vi "teleop.vi"() -> ()   [LabVIEW 2012, in "Team8953.lvrbt"]
uses:
  Team8953.lvrbt
  <vilib>/NXT/Hardware/Plugins/Tetrix 180 deg Servo/Tetrix180ServoAddress.ctl
  <vilib>/NXT/Hardware/Plugins/Tetrix DC Motor/TetrixDCMotorAddress.ctl
  <vilib>/FTC/FTC Read Controller Packet.vi
  <vilib>/FTC/FTC Read Button States.vi
  <vilib>/NXT/NXTIO Xnodes/NXTIONodeSubVIs/TETRIX IO Move Servos.vi
  <vilib>/FTC/FTC Calculate Drive Power - Arcade Right.vi
  <vilib>/NXT/NXTIO Xnodes/NXTIONodeSubVIs/TETRIX IO Move DC Motors.vi
  <vilib>/NXT/NXTIO Xnodes/NXTIONodeSubVIs/TETRIX IO Check Battery.vi
  <vilib>/NXT/NXTIO Xnodes/NXTIONodeSubVIs/TETRIX IO Stop DC Motors.vi
  <vilib>/NXT/Subs/LVHSConnector.ctl
  <vilib>/NXT/NXTIO Xnodes/AddressXNode/NXTIOAddress.xnode
  <vilib>/NXT/NXTIO Xnodes/NXTIOXNode/NXTIO.xnode
  <vilib>/NXT/LegoClasses/BrickReference/BrickReference.lvclass
panel:
  in  "Drive Power":i8=100 min=-100 max=100
  # "This VI was generated based on your configuration in the Remote Control Editor. You may modify the code as needed for your robot. To test this program for an FTC match, return to the Remote Control Editor, select the \"Run Program\" tab, and choose \"Teleop\"."
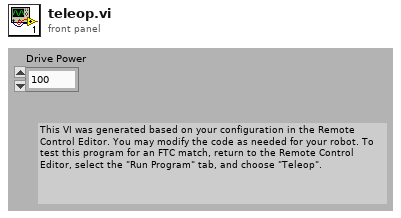
[diagram p1: front panel]
types:
  T1 = typedef "TetrixDCMotorAddress.ctl" = i32
  T2 = cluster{"TetrixDCMotor":T1, "TetrixDCMotor 2":T1}
  T3 = typedef "LVHSConnector.ctl" = refnum<class "BrickReference.lvclass">
  T4 = typedef "FTC ControllerState.ctl" = cluster{"Left X":i8, "Left Y":i8, "Right X":i8, "Right Y":i8, "Button Encoding 9-12":u8, "Button Encoding 1-8":u8, "POV":T5}
  T5 = typedef "FTC POVState.ctl" = i8
  T6 = typedef "FTC ButtonEventType.ctl" = enum16{"Pressed", "Released"}
  T7 = cluster{"Button ID":enum16{"None", "Button 1", "Button 2", "Button 3", "Button 4", "Button 5", "Button 6", "Button 7", "Button 8", "Button 9", "Button 10", "Button 11", "Button 12", "POV Up", "POV Up Right", "POV Right", "POV Down Right", "POV Down", "POV Down Left", "POV Left", "POV Up Left"}, "Event Type":T6}[]
  T8 = enum16{"None", "Button 1", "Button 2", "Button 3", "Button 4", "Button 5", "Button 6", "Button 7", "Button 8", "Button 9", "Button 10", "Button 11", "Button 12", "POV Up", "POV Up Right", "POV Right", "POV Down Right", "POV Down", "POV Down Left", "POV Left", "POV Up Left"}
  T9 = typedef "Tetrix180ServoAddress.ctl" = i32
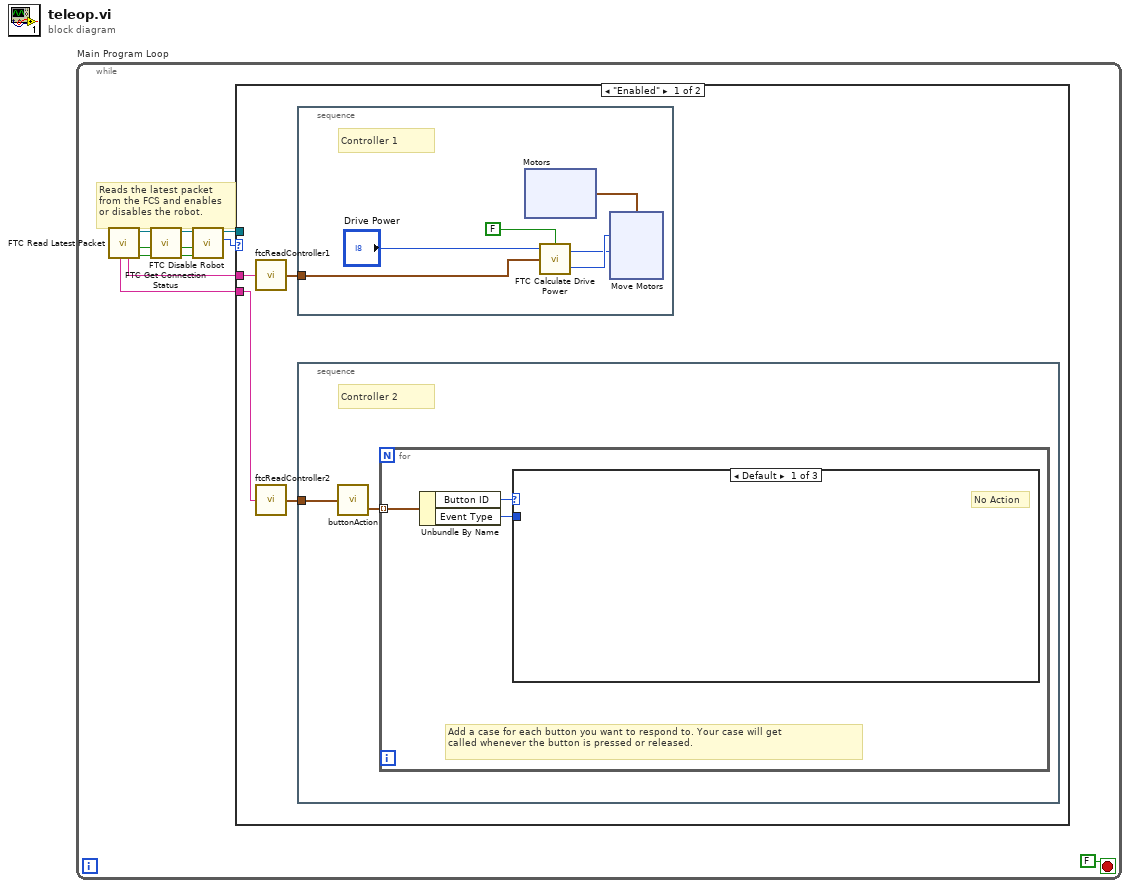
[diagram p0: block diagram]
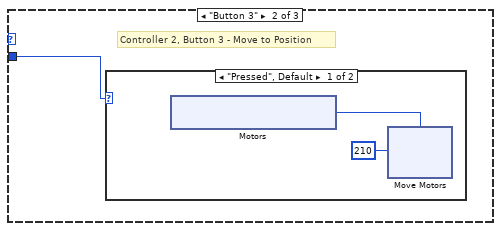
[diagram p2: hidden frame]
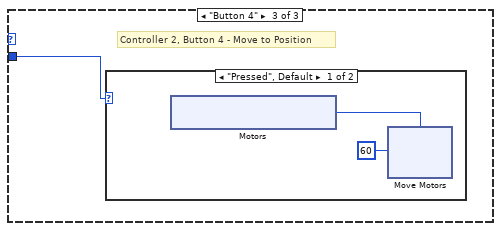
[diagram p4: hidden frame]
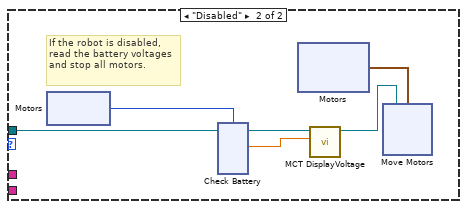
[diagram p6: hidden frame]
diagram:
  n1 = while "Main Program Loop" {
    stop <- FALSE stop-if-true
    # "Reads the latest packet\nfrom the FCS and enables\nor disables the robot."
    n2 = call <vilib>:"FTC Read Latest Packet.vi"() -> ("Packet Received?"=w8:bool, "Stopped?"=w5:bool, "NXT/EV3"=w7:T3, "Controller 1"=w10:string, "Controller 2"=w9:string)  [unwired: 6 in, 1 out]
    n3 = call <vilib>:"FTC Get Connection Status.vi"("Packet Received?"=w8, "Stopped?"=w5, "NXT/EV3"=w7) -> ("Online?"=w2:bool, "Stopped?"=w3:bool, "NXT/EV3"=w4:T3)  [unwired: 5 in]
    n4 = call <vilib>:"FTC Disable Robot.vi"("Online?"=w2, "Stopped?"=w3, "NXT/EV3"=w4) -> ("Enabled?"=w6:enum16{"Disabled", "Enabled"}, "NXT/EV3"=w1:T3)  [unwired: 3 in]
    n5 = case "disableCase" shown="\"Enabled\"" w6 {
      tunnel: w10 -> [w15 _]
      tunnel: w9 -> [w14 _]
      tunnel: w1 -> [_ w63]
      frame "Enabled" {
        n6 = call "ftcReadController1"("Packet"=w15) -> ("Controller State"=w13:T4)  [unwired: 4 in]
        n7 = call "ftcReadController2"("Packet"=w14) -> ("Controller State"=w12:T4)  [unwired: 4 in]
        n8 = stacked-sequence "controller1Actions" {
          tunnel: w13 -> [w48]
          frame #0 {
            # "Controller 1"
            n9 = xnode ("Motors")() -> ("Motor"=w45:cluster{"TetrixDCMotor":T1, "TetrixDCMotor":T1})
            n10 = call-poly <vilib>:"FTC Calculate Drive Power.vi"("Reverse"=FALSE, "Controller State"=w48, "Power Level (50)"="Drive Power") -> ("Right Motor Power"=w44:i8, "Left Motor Power"=w43:i8)  [unwired: 1 in]
            n11 = xnode ("Move Motors")("Power/Speed 2"=w43, "Power/Speed 1"=w44, "Motors"=w45) -> ()  [unwired: 1 in, 1 out]
          }
        }
        n12 = stacked-sequence "controller2Actions" {
          tunnel: w12 -> [w16]
          frame #0 {
            # "Controller 2"
            n13 = call "buttonAction"("Controller State"=w16) -> ("Button Events"=w17:T7)  [unwired: 2 in, 1 out]
            n14 = for "buttonAction" {
              tunnel: w17 -> [w18] mode=indexing
              # "Add a case for each button you want to respond to. Your case will get \ncalled whenever the button is pressed or released."
              n15 = Unbundle By Name(w18) -> ("Button ID"=w20:T8, "Event Type"=w19:T6)
              n16 = case "EventCase2" shown="Default" w20 {
                tunnel: w19 -> [_ w21 w32]
                frame Default {
                  # "No Action"
                }
                frame "Button 3" {
                  # "Controller 2, Button 3 - Move to Position"
                  n17 = case shown="\"Pressed\", Default" w21 {
                    frame "Pressed", Default {
                      n18 = xnode "Motors"() -> ("Motor"=w23:T9)
                      n19 = xnode "Move Motors"("Position 1"=210, "Motors"=w23) -> ()  [unwired: 1 in, 1 out]
                    }
                    frame "Released" {
                    }
                  }
                }
                frame "Button 4" {
                  # "Controller 2, Button 4 - Move to Position"
                  n20 = case shown="\"Pressed\", Default" w32 {
                    frame "Pressed", Default {
                      n21 = xnode "Motors"() -> ("Motor"=w34:T9)
                      n22 = xnode "Move Motors"("Position 1"=60, "Motors"=w34) -> ()  [unwired: 1 in, 1 out]
                    }
                    frame "Released" {
                    }
                  }
                }
              }
            }
          }
        }
      }
      frame "Disabled" {
        # "If the robot is disabled, read the battery voltages and stop all motors."
        n23 = xnode ("Motors")() -> ("Motor"=w62:T1)
        n24 = xnode ("Check Battery")("Motors"=w62, "NXT/EV3"=w63) -> ("Voltage 1"=w61:sgl, "NXT/EV3"=w60:T3)
        n25 = xnode "Motors"() -> ("Motor"=w59:cluster{"TetrixDCMotor":T1, "TetrixDCMotor":T1})
        n26 = call <vilib>:"MCT DisplayVoltage.vi"("Motor Voltage"=w61, "NXT/EV3"=w60) -> ("NXT/EV3"=w58:T3)  [unwired: 9 in]
        n27 = xnode "Move Motors"("Motors"=w59, "NXT/EV3"=w58) -> ()  [unwired: 1 out]
      }
    }
  }
